vi "Set(path).vi"(8 "error in (no error)":errorcluster, 9 "value to set":refnum<class "JSON Value.lvclass">, 10 "Path":string, 11 "JSON Value in":refnum<class "JSON Value.lvclass">) -> (0 "error out":errorcluster, 3 "JSON Value out":refnum<class "JSON Value.lvclass">)   [LabVIEW 2016, in "JSON Value.lvclass"]
uses:
  JSON Value.lvclass
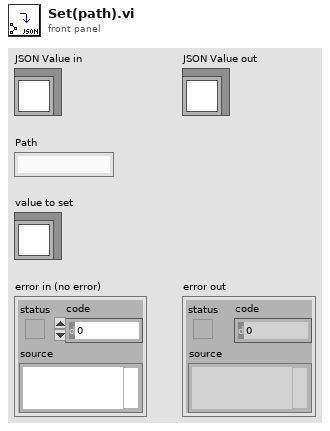
[diagram p1: front panel]
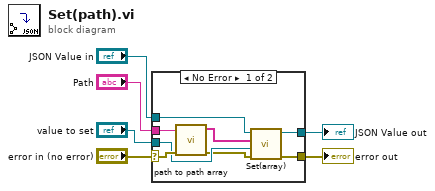
[diagram p0: block diagram]
diagram:
  n1 = case shown="No Error" "error in (no error)" {
    selector: "error in (no error)" -> [w14 w15]
    tunnel: [w7 w16] -> w4
    tunnel: "JSON Value in" -> [w11 w16]
    tunnel: "Path" -> [w13 _]
    tunnel: "value to set" -> [w10 _]
    tunnel: [w9 w15] -> w1
    frame No Error {
      n2 = call "path to path array.vi"("error in (no error)"=w14, "path"=w13) -> ("error out"=w8:errorcluster, "path array"=w12:string[])  [unwired: 8 in]
      n3 = call "Set(array).vi"("error in (no error)"=w8, "value to set"=w10, "Path Array"=w12, "JSON Value in"=w11) -> ("error out"=w9:errorcluster, "JSON Value out"=w7:refnum<class "JSON Value.lvclass">)  [unwired: 6 in]
    }
    frame Error {
    }
  }
  "error out" <- w1
  "JSON Value out" <- w4
